vi "ParamScanSubVI.vi"(7 "Variable Cluster":T1={"Values"=[105.34210526315789, 210.5842105263158, 315.8263157894737, 421.0684210526316, 26.410526315789475, 131.65263157894736, 236.89473684210526, 342.1368421052632, 447.3789473684211, 52.72105263157895, 157.96315789473684, 263.20526315789476, 368.44736842105266, 473.68947368421055, 79.03157894736842, 184.2736842105263, 289.5157894736842, 394.7578947368421, 500.0], "Action"=20, "Inst."=0, "# Elements"=20, "Next Element"=6, "First Val"=0.1, "Final Val"=500.0, "Update Array"=FALSE, "Description"="relax", "Variable Type"=0, "Scan Now"=FALSE, "# Act/Inst."=11, "Electrodes_range"=[], "Parameter Name"="RW frequency (Hz)", "# Passes"=4} {"Variable Type" items=["Duration (s)", "Voltage (V)", "Parameter"]; "Final Val" format="%_6p"; "First Val" format="%_6p"; "Values" format="%_6p"}, 8 "Actions in":T4=[{"Toggle"=TRUE, "Open parameter editor"=FALSE, "Open MacroEditor"=FALSE, "Macro path"=path "", "Duration (s)"=2.0, "Parameters"=[{"Status"="Camera", "Name"="state (0,1)", "Value"=0.0, "Changed"=FALSE}, {"Status"="Slave", "Name"="state (0,1)", "Value"=0.0, "Changed"=FALSE}, {"Status"="Wait", "Name"="inbit (0...7)", "Value"=0.0, "Changed"=FALSE}, {"Status"="Coils", "Name"="buncher (A)", "Value"=10.0, "Changed"=TRUE}, {"Status"="Coils", "Name"="exit (A)", "Value"=25.0, "Changed"=TRUE}, {"Status"="Coils", "Name"="source (A)", "Value"=0.0, "Changed"=FALSE}, {"Status"="Coils", "Name"="stacker (A)", "Value"=0.0, "Changed"=FALSE}, {"Status"="Coils", "Name"="trans2 (A)", "Value"=0.0, "Changed"=FALSE}, {"Status"="Coils", "Name"="trans3 (A)", "Value"=0.0, "Changed"=FALSE}, {"Status"="Coils", "Name"="trans4 (A)", "Value"=0.0, "Changed"=FALSE}, {"Status"="RW", "Name"="mode (0-9)", "Value"=0.0, "Changed"=FALSE}, {"Status"="RW", "Name"="f_start (Hz)", "Value"=0.0, "Changed"=FALSE}, {"Status"="RW", "Name"="f_stop (Hz)", "Value"=0.0, "Changed"=FALSE}, {"Status"="RW", "Name"="amplitude (V)", "Value"=0.0, "Changed"=FALSE}, {"Status"="RW", "Name"="phase dif (deg)", "Value"=0.0, "Changed"=FALSE}, {"Status"="RW", "Name"="sweep time (s)", "Value"=0.0, "Changed"=FALSE}, {"Status"="HVpuls1", "Name"="enable (0,1)", "Value"=0.0, "Changed"=FALSE}, {"Status"="HVpuls1", "Name"="amplitude (V)", "Value"=0.0, "Changed"=FALSE}, {"Status"="HVpuls2", "Name"="enable (0,1)", "Value"=0.0, "Changed"=FALSE}, {"Status"="HVpuls2", "Name"="amplitude (V)", "Value"=0.0, "Changed"=FALSE}, {"Status"="HVpuls3", "Name"="enable (0,1)", "Value"=0.0, "Changed"=FALSE}, {"Status"="HVpuls3", "Name"="amplitude (V)", "Value"=0.0, "Changed"=FALSE}, {"Status"="MCP", "Name"="front bias (V)", "Value"=0.0, "Changed"=FALSE}, {"Status"="MCP", "Name"="back bias (V)", "Value"=0.0, "Changed"=FALSE}, {"Status"="MCP", "Name"="phos bias (V)", "Value"=0.0, "Changed"=FALSE}], "Comment"="buncher and exit on", "Reps"=1}, {"Toggle"=TRUE, "Open parameter editor"=FALSE, "Open MacroEditor"=FALSE, "Macro path"=path "", "Duration (s)"=0.1, "Parameters"=[{"Status"="Camera", "Name"="state (0,1)", "Value"=0.0, "Changed"=FALSE}, {"Status"="Slave", "Name"="state (0,1)", "Value"=0.0, "Changed"=FALSE}, {"Status"="Wait", "Name"="inbit (0...7)", "Value"=0.0, "Changed"=FALSE}, {"Status"="Coils", "Name"="buncher (A)", "Value"=0.0, "Changed"=TRUE}, {"Status"="Coils", "Name"="exit (A)", "Value"=0.0, "Changed"=TRUE}, {"Status"="Coils", "Name"="source (A)", "Value"=0.0, "Changed"=FALSE}, {"Status"="Coils", "Name"="stacker (A)", "Value"=0.0, "Changed"=FALSE}, {"Status"="Coils", "Name"="trans2 (A)", "Value"=0.0, "Changed"=FALSE}, {"Status"="Coils", "Name"="trans3 (A)", "Value"=0.0, "Changed"=FALSE}, {"Status"="Coils", "Name"="trans4 (A)", "Value"=0.0, "Changed"=FALSE}, {"Status"="RW", "Name"="mode (0-9)", "Value"=0.0, "Changed"=FALSE}, {"Status"="RW", "Name"="f_start (Hz)", "Value"=0.0, "Changed"=FALSE}, {"Status"="RW", "Name"="f_stop (Hz)", "Value"=0.0, "Changed"=FALSE}, {"Status"="RW", "Name"="amplitude (V)", "Value"=0.0, "Changed"=FALSE}, {"Status"="RW", "Name"="phase dif (deg)", "Value"=0.0, "Changed"=FALSE}, {"Status"="RW", "Name"="sweep time (s)", "Value"=0.0, "Changed"=FALSE}, {"Status"="HVpuls1", "Name"="enable (0,1)", "Value"=0.0, "Changed"=FALSE}, {"Status"="HVpuls1", "Name"="amplitude (V)", "Value"=0.0, "Changed"=FALSE}, {"Status"="HVpuls2", "Name"="enable (0,1)", "Value"=0.0, "Changed"=FALSE}, {"Status"="HVpuls2", "Name"="amplitude (V)", "Value"=0.0, "Changed"=FALSE}, {"Status"="HVpuls3", "Name"="enable (0,1)", "Value"=0.0, "Changed"=FALSE}, {"Status"="HVpuls3", "Name"="amplitude (V)", "Value"=0.0, "Changed"=FALSE}, {"Status"="MCP", "Name"="front bias (V)", "Value"=0.0, "Changed"=FALSE}, {"Status"="MCP", "Name"="back bias (V)", "Value"=0.0, "Changed"=FALSE}, {"Status"="MCP", "Name"="phos bias (V)", "Value"=0.0, "Changed"=FALSE}], "Comment"="off", "Reps"=1}] {"Reps" min=1 step=1; "Parameters"."Value" format="%_6p"; "Duration (s)" min=0.001 step=0.001 format="%_6p"}, 9 "Macro Info 2D in":T2(array[cluster])=[[{"Duration (s)"=2.0, "Instruction Description"="buncher and exit on", "Input Bits"=[], "Output Bits"=[FALSE, FALSE, FALSE, FALSE, FALSE, FALSE, FALSE, FALSE, FALSE, FALSE, FALSE, FALSE, FALSE, FALSE, FALSE, FALSE, FALSE, FALSE, FALSE, FALSE, FALSE, FALSE, FALSE, FALSE, FALSE, FALSE, FALSE, FALSE, FALSE, FALSE, FALSE, FALSE, FALSE, FALSE, FALSE, FALSE, FALSE, FALSE], "Excitations"=[0.0, 0.0, 0.0, 0.0, 0.0, 0.0, 0.0, 0.0, 0.0, 0.0, 0.0, 0.0, 0.0, 0.0, 0.0, 0.0, 0.0, 0.0, 0.0, 0.0, 0.0, 0.0, 0.0, 0.0], "Steps"=1, "Changes"=[TRUE, TRUE]}], [{"Duration (s)"=0.1, "Instruction Description"="off", "Input Bits"=[], "Output Bits"=[FALSE, FALSE, FALSE, FALSE, FALSE, FALSE, FALSE, FALSE, FALSE, FALSE, FALSE, FALSE, FALSE, FALSE, FALSE, FALSE, FALSE, FALSE, FALSE, FALSE, FALSE, FALSE, FALSE, FALSE, FALSE, FALSE, FALSE, FALSE, FALSE, FALSE, FALSE, FALSE, FALSE, FALSE, FALSE, FALSE, FALSE, FALSE], "Excitations"=[0.0, 0.0, 0.0, 0.0, 0.0, 0.0, 0.0, 0.0, 0.0, 0.0, 0.0, 0.0, 0.0, 0.0, 0.0, 0.0, 0.0, 0.0, 0.0, 0.0, 0.0, 0.0, 0.0, 0.0], "Steps"=1, "Changes"=[TRUE, TRUE]}]], 10 "# always zero":i32, 11 "Calibrations":T3=[{"Gain"=15.0098, "Offset (V)"=0.0035, "Name"="Vm"}, {"Gain"=14.9932, "Offset (V)"=0.0066, "Name"="in"}, {"Gain"=14.9651, "Offset (V)"=0.0072, "Name"="s1"}, {"Gain"=14.9843, "Offset (V)"=0.0049, "Name"="s2"}, {"Gain"=14.9433, "Offset (V)"=0.0056, "Name"="s3"}, {"Gain"=14.9395, "Offset (V)"=0.0041, "Name"="s4"}, {"Gain"=14.8775, "Offset (V)"=0.006, "Name"="g8"}, {"Gain"=14.9361, "Offset (V)"=0.0045, "Name"="--"}, {"Gain"=15.1086, "Offset (V)"=0.0054, "Name"="e1"}, {"Gain"=14.9264, "Offset (V)"=0.0039, "Name"="c1"}, {"Gain"=14.8685, "Offset (V)"=0.0066, "Name"="c2"}, {"Gain"=14.9386, "Offset (V)"=0.0045, "Name"="c3"}, {"Gain"=14.9438, "Offset (V)"=0.0032, "Name"="c4"}, {"Gain"=14.93, "Offset (V)"=0.0052, "Name"="c5"}, {"Gain"=14.9119, "Offset (V)"=0.0093, "Name"="c6"}, {"Gain"=14.9135, "Offset (V)"=0.0055, "Name"="c7"}, {"Gain"=14.9961, "Offset (V)"=0.0148, "Name"="c8"}, {"Gain"=14.9315, "Offset (V)"=0.0024, "Name"="c9"}, {"Gain"=14.9245, "Offset (V)"=0.006, "Name"="e2"}, {"Gain"=14.9016, "Offset (V)"=0.0037, "Name"="--"}, {"Gain"=14.9057, "Offset (V)"=0.0055, "Name"="--"}, {"Gain"=14.9213, "Offset (V)"=0.004, "Name"="--"}, {"Gain"=14.8995, "Offset (V)"=0.0013, "Name"="--"}, {"Gain"=14.9373, "Offset (V)"=0.004, "Name"="--"}] {"Offset (V)" format="%_6p"; "Gain" format="%_6p"}) -> (0 "Actions out":T4=[{"Toggle"=TRUE, "Open parameter editor"=FALSE, "Open MacroEditor"=FALSE, "Macro path"=path "", "Duration (s)"=2.0, "Parameters"=[{"Status"="Camera", "Name"="state (0,1)", "Value"=0.0, "Changed"=FALSE}, {"Status"="Slave", "Name"="state (0,1)", "Value"=0.0, "Changed"=FALSE}, {"Status"="Wait", "Name"="inbit (0...7)", "Value"=0.0, "Changed"=FALSE}, {"Status"="Coils", "Name"="buncher (A)", "Value"=10.0, "Changed"=TRUE}, {"Status"="Coils", "Name"="exit (A)", "Value"=30.0, "Changed"=TRUE}, {"Status"="Coils", "Name"="source (A)", "Value"=0.0, "Changed"=FALSE}, {"Status"="Coils", "Name"="stacker (A)", "Value"=0.0, "Changed"=FALSE}, {"Status"="Coils", "Name"="trans2 (A)", "Value"=0.0, "Changed"=FALSE}, {"Status"="Coils", "Name"="trans3 (A)", "Value"=0.0, "Changed"=FALSE}, {"Status"="Coils", "Name"="trans4 (A)", "Value"=0.0, "Changed"=FALSE}, {"Status"="RW", "Name"="mode (0-9)", "Value"=0.0, "Changed"=FALSE}, {"Status"="RW", "Name"="f_start (Hz)", "Value"=0.0, "Changed"=FALSE}, {"Status"="RW", "Name"="f_stop (Hz)", "Value"=0.0, "Changed"=FALSE}, {"Status"="RW", "Name"="amplitude (V)", "Value"=0.0, "Changed"=FALSE}, {"Status"="RW", "Name"="phase dif (deg)", "Value"=0.0, "Changed"=FALSE}, {"Status"="RW", "Name"="sweep time (s)", "Value"=0.0, "Changed"=FALSE}, {"Status"="HVpuls1", "Name"="enable (0,1)", "Value"=0.0, "Changed"=FALSE}, {"Status"="HVpuls1", "Name"="amplitude (V)", "Value"=0.0, "Changed"=FALSE}, {"Status"="HVpuls2", "Name"="enable (0,1)", "Value"=0.0, "Changed"=FALSE}, {"Status"="HVpuls2", "Name"="amplitude (V)", "Value"=0.0, "Changed"=FALSE}, {"Status"="HVpuls3", "Name"="enable (0,1)", "Value"=0.0, "Changed"=FALSE}, {"Status"="HVpuls3", "Name"="amplitude (V)", "Value"=0.0, "Changed"=FALSE}, {"Status"="MCP", "Name"="front bias (V)", "Value"=0.0, "Changed"=FALSE}, {"Status"="MCP", "Name"="back bias (V)", "Value"=0.0, "Changed"=FALSE}, {"Status"="MCP", "Name"="phos bias (V)", "Value"=0.0, "Changed"=FALSE}], "Comment"="buncher and exit on", "Reps"=1}, {"Toggle"=TRUE, "Open parameter editor"=FALSE, "Open MacroEditor"=FALSE, "Macro path"=path "", "Duration (s)"=0.1, "Parameters"=[{"Status"="Camera", "Name"="state (0,1)", "Value"=0.0, "Changed"=FALSE}, {"Status"="Slave", "Name"="state (0,1)", "Value"=0.0, "Changed"=FALSE}, {"Status"="Wait", "Name"="inbit (0...7)", "Value"=0.0, "Changed"=FALSE}, {"Status"="Coils", "Name"="buncher (A)", "Value"=0.0, "Changed"=TRUE}, {"Status"="Coils", "Name"="exit (A)", "Value"=0.0, "Changed"=TRUE}, {"Status"="Coils", "Name"="source (A)", "Value"=0.0, "Changed"=FALSE}, {"Status"="Coils", "Name"="stacker (A)", "Value"=0.0, "Changed"=FALSE}, {"Status"="Coils", "Name"="trans2 (A)", "Value"=0.0, "Changed"=FALSE}, {"Status"="Coils", "Name"="trans3 (A)", "Value"=0.0, "Changed"=FALSE}, {"Status"="Coils", "Name"="trans4 (A)", "Value"=0.0, "Changed"=FALSE}, {"Status"="RW", "Name"="mode (0-9)", "Value"=0.0, "Changed"=FALSE}, {"Status"="RW", "Name"="f_start (Hz)", "Value"=0.0, "Changed"=FALSE}, {"Status"="RW", "Name"="f_stop (Hz)", "Value"=0.0, "Changed"=FALSE}, {"Status"="RW", "Name"="amplitude (V)", "Value"=0.0, "Changed"=FALSE}, {"Status"="RW", "Name"="phase dif (deg)", "Value"=0.0, "Changed"=FALSE}, {"Status"="RW", "Name"="sweep time (s)", "Value"=0.0, "Changed"=FALSE}, {"Status"="HVpuls1", "Name"="enable (0,1)", "Value"=0.0, "Changed"=FALSE}, {"Status"="HVpuls1", "Name"="amplitude (V)", "Value"=0.0, "Changed"=FALSE}, {"Status"="HVpuls2", "Name"="enable (0,1)", "Value"=0.0, "Changed"=FALSE}, {"Status"="HVpuls2", "Name"="amplitude (V)", "Value"=0.0, "Changed"=FALSE}, {"Status"="HVpuls3", "Name"="enable (0,1)", "Value"=0.0, "Changed"=FALSE}, {"Status"="HVpuls3", "Name"="amplitude (V)", "Value"=0.0, "Changed"=FALSE}, {"Status"="MCP", "Name"="front bias (V)", "Value"=0.0, "Changed"=FALSE}, {"Status"="MCP", "Name"="back bias (V)", "Value"=0.0, "Changed"=FALSE}, {"Status"="MCP", "Name"="phos bias (V)", "Value"=0.0, "Changed"=FALSE}], "Comment"="off", "Reps"=1}] {"Reps" min=1 step=1; "Parameters"."Value" format="%_6p"; "Duration (s)" min=0.001 step=0.001 format="%_6p"}, 1 "Macro Info 2D out":T2(array[cluster])=[[{"Duration (s)"=2.0, "Instruction Description"="buncher and exit on", "Input Bits"=[], "Output Bits"=[FALSE, FALSE, FALSE, FALSE, FALSE, FALSE, FALSE, FALSE, FALSE, FALSE, FALSE, FALSE, FALSE, FALSE, FALSE, FALSE, FALSE, FALSE, FALSE, FALSE, FALSE, FALSE, FALSE, FALSE, FALSE, FALSE, FALSE, FALSE, FALSE, FALSE, FALSE, FALSE, FALSE, FALSE, FALSE, FALSE, FALSE, FALSE], "Excitations"=[0.0, 0.0, 0.0, 0.0, 0.0, 0.0, 0.0, 0.0, 0.0, 0.0, 0.0, 0.0, 0.0, 0.0, 0.0, 0.0, 0.0, 0.0, 0.0, 0.0, 0.0, 0.0, 0.0, 0.0], "Steps"=1, "Changes"=[TRUE, TRUE]}], [{"Duration (s)"=0.1, "Instruction Description"="off", "Input Bits"=[], "Output Bits"=[FALSE, FALSE, FALSE, FALSE, FALSE, FALSE, FALSE, FALSE, FALSE, FALSE, FALSE, FALSE, FALSE, FALSE, FALSE, FALSE, FALSE, FALSE, FALSE, FALSE, FALSE, FALSE, FALSE, FALSE, FALSE, FALSE, FALSE, FALSE, FALSE, FALSE, FALSE, FALSE, FALSE, FALSE, FALSE, FALSE, FALSE, FALSE], "Excitations"=[0.0, 0.0, 0.0, 0.0, 0.0, 0.0, 0.0, 0.0, 0.0, 0.0, 0.0, 0.0, 0.0, 0.0, 0.0, 0.0, 0.0, 0.0, 0.0, 0.0, 0.0, 0.0, 0.0, 0.0], "Steps"=1, "Changes"=[TRUE, TRUE]}]])   [LabVIEW 2018]
uses:
  QBuilder Files/Actions_arr.ctl
  QBuilder Files/Action.ctl
  QBuilder Files/Parameters.ctl
  Calibrations.ctl
  VariableScan_Cluster.ctl
panel:
  # "browse"
  # "browse"
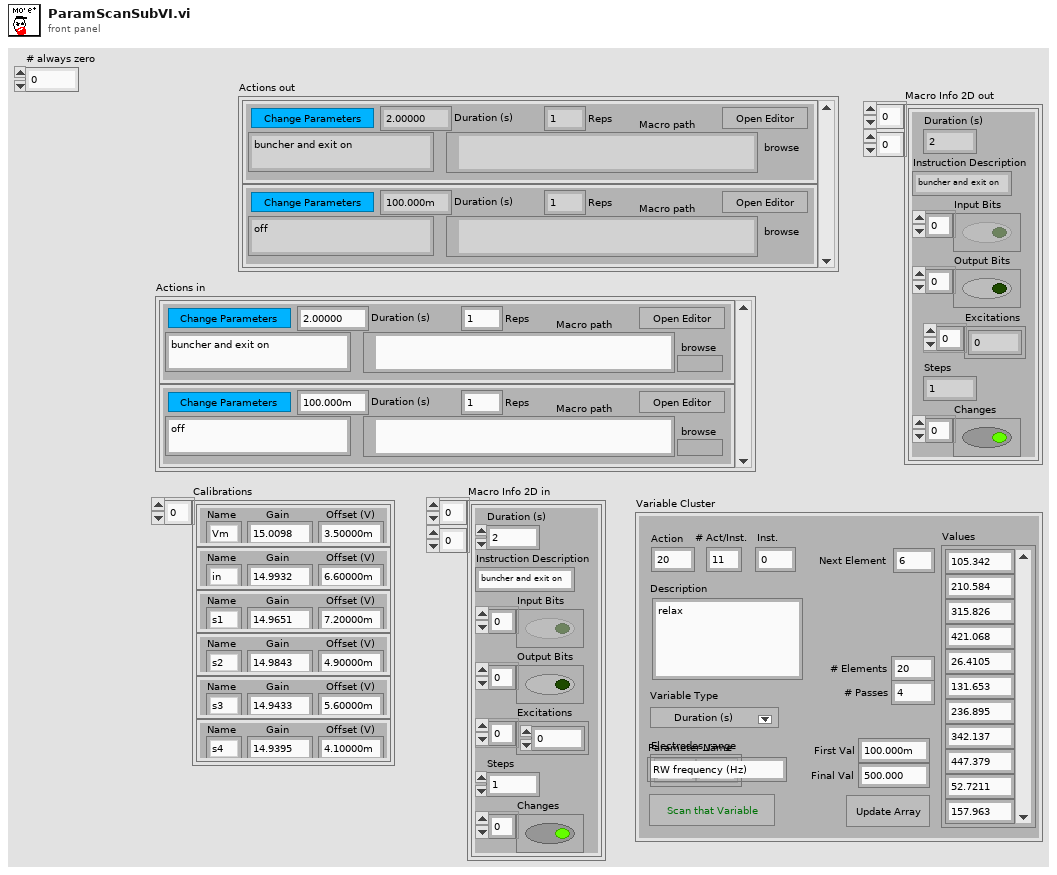
[diagram p1: front panel]
types:
  T1 = typedef "VariableScan_Cluster.ctl" = cluster{"Values":dbl[], "Action":i32, "Inst.":i32, "# Elements":i32, "Next Element":i32, "First Val":dbl, "Final Val":dbl, "Update Array":bool, "Description":string, "Variable Type":u16, "Scan Now":bool, "# Act/Inst.":i32, "Electrodes_range":i32[], "Parameter Name":string, "# Passes":i32}
  T2 = cluster{"Duration (s)":dbl, "Instruction Description":string, "Input Bits":bool[], "Output Bits":bool[], "Excitations":dbl[], "Steps":i32, "Changes":bool[]}[][]
  T3 = typedef "Calibrations.ctl" = cluster{"Gain":dbl, "Offset (V)":dbl, "Name":string}[]
  T4 = typedef "Actions_arr.ctl" = T5[]
  T5 = typedef "Action.ctl" = cluster{"Toggle":bool, "Open parameter editor":bool, "Open MacroEditor":bool, "Macro path":path, "Duration (s)":dbl, "Parameters":T6, "Comment":string, "Reps":i32}
  T6 = typedef "Parameters.ctl" = cluster{"Status":string, "Name":string, "Value":dbl, "Changed":bool}[]
  T7 = cluster{"Duration (s)":dbl, "Instruction Description":string, "Input Bits":bool[], "Output Bits":bool[], "Excitations":dbl[], "Steps":i32, "Changes":bool[]}
  T8 = cluster{"Status":string, "Name":string, "Value":dbl, "Changed":bool}
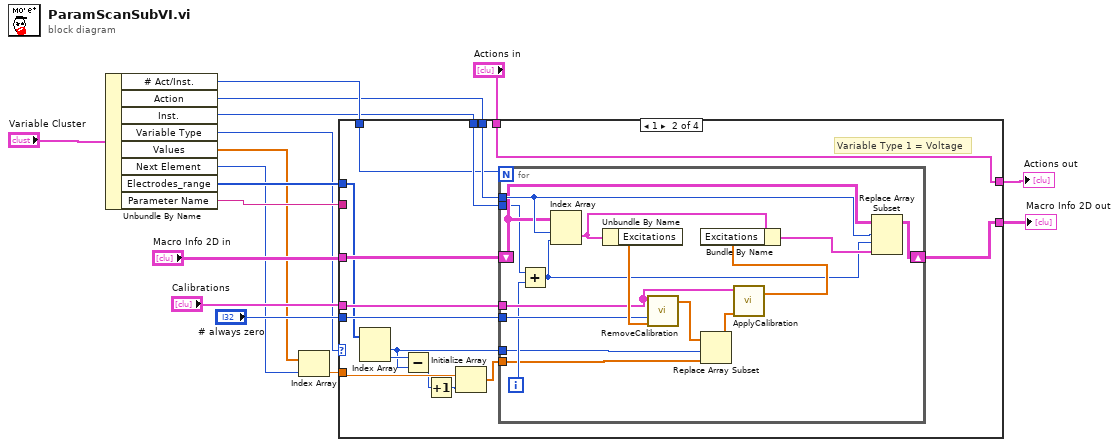
[diagram p0: block diagram]
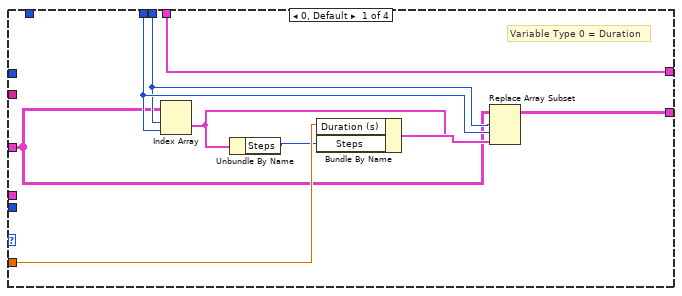
[diagram p2: hidden frame]
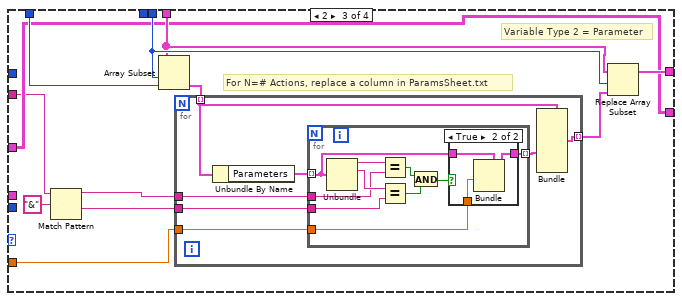
[diagram p3: hidden frame]
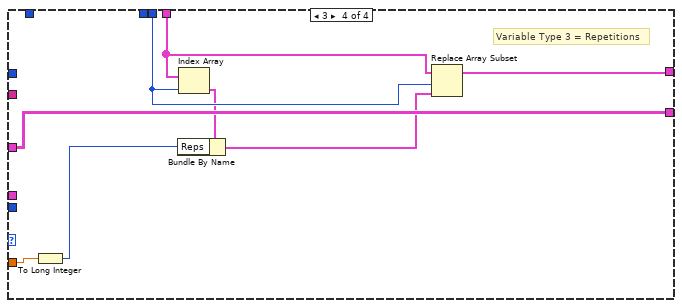
[diagram p5: hidden frame]
diagram:
  n1 = Unbundle By Name("Variable Cluster") -> ("# Act/Inst."=w8:i32, "Action"=w3:i32, "Inst."=w4:i32, "Variable Type"=w6:u16, "Values"=w7:dbl[], "Next Element"=w1:i32, "Electrodes_range"=w10:i32[], "Parameter Name"=w9:string)
  n2 = Index Array(array=w7, index=w1) -> (element=w5:dbl)
  n3 = case shown="1" w6 {
    tunnel: w3 -> [w22 w40 w68 w94]
    tunnel: w4 -> [w25 w39 _ _]
    tunnel: w5 -> [w21 w32 w57 w97]
    tunnel: w8 -> [_ w33 w65 _]
    tunnel: w9 -> [_ _ w60 _]
    tunnel: w10 -> [_ w30 _ _]
    tunnel: "Macro Info 2D in" -> [w19 w37 w62 w96]
    tunnel: [w18 w38 w62 w96] -> w12
    tunnel: "Calibrations" -> [_ w36 _ _]
    tunnel: "# always zero" -> [_ w35 _ _]
    tunnel: "Actions in" -> [w17 w34 w64 w95]
    tunnel: [w17 w34 w63 w90] -> w16
    frame 0, Default {
      # "Variable Type 0 = Duration"
      n4 = Index Array(array=w19, index (row)=w22, index (col)=w25) -> (element=w23:T7)
      n5 = Unbundle By Name(w23) -> ("Steps"=w20:i32)
      n6 = Bundle By Name(cluster=w23, "Duration (s)"=w21, "Steps"=w20) -> (w24:T7)
      n7 = Replace Array Subset(array=w19, new element=w24, index (row)=w22, index (col)=w25) -> (w18:T2)
    }
    frame 1 {
      # "Variable Type 1 = Voltage"
      n8 = Index Array(array=w30) -> (element #1=w28:i32, element #2=w29:i32)  [unwired: 2 in]
      n9 = Subtract(x=w29, y=w28) -> (x-y=w27:i32)
      n10 = Increment(x=w27) -> (x+1=w26:i32)
      n11 = Initialize Array(w32, w26) -> (w31:dbl[])
      n12 = for {
        N: w33 -> [_]
        tunnel: w40 -> [w55]
        tunnel: w39 -> [w45]
        tunnel: w36 -> [w47]
        tunnel: w35 -> [w46]
        shift-right: [w49] -> w38
        shift-left: w37 -> [w48]
        tunnel: w31 -> [w42]
        tunnel: w28 -> [w41]
        i -> [w44]
        n13 = Add(x=w45, y=w44) -> (x+y=w43:i32)
        n14 = Index Array(array=w48, index (row)=w55, index (col)=w43) -> (element=w56:T7)
        n15 = Unbundle By Name(w56) -> ("Excitations"=w53:dbl[])
        n16 = call "RemoveCalibration.vi"("Excitations"=w53, "# always zero"=w46, "Calibrations"=w47) -> ("Potentials"=w52:dbl[])  [unwired: 2 in]
        n17 = Replace Array Subset(array=w52, new element=w42, index=w41) -> (w51:dbl[])
        n18 = call "ApplyCalibration.vi"("Potentials"=w51, "Calibrations"=w47) -> ("Excitations"=w50:dbl[])  [unwired: 2 in, 1 out]
        n19 = Bundle By Name(cluster=w56, "Excitations"=w50) -> (w54:T7)
        n20 = Replace Array Subset(array=w48, new element=w54, index (row)=w55, index (col)=w43) -> (w49:T2)
      }
    }
    frame 2 {
      # "For N=# Actions, replace a column in ParamsSheet.txt"
      # "Variable Type 2 = Parameter"
      n21 = Match Pattern(string=w60, regular expression="&") -> (before substring=w59:string, after substring=w58:string)  [unwired: 1 in, 2 out]
      n22 = Array Subset(array=w64, index=w68, length=w65) -> (w67:T4)
      n23 = for {
        tunnel: w57 -> [w75]
        tunnel: w67 -> [w72] mode=indexing
        tunnel: [w71] -> w66 mode=indexing
        tunnel: w59 -> [w70]
        tunnel: w58 -> [w69]
        n24 = Unbundle By Name(w72) -> ("Parameters"=w73:T6)
        n25 = for {
          tunnel: w73 -> [w85] mode=indexing
          tunnel: [w84] -> w74 mode=indexing
          tunnel: w75 -> [w83]
          tunnel: w70 -> [w77]
          tunnel: w69 -> [w76]
          n26 = Unbundle(w85) -> ("Status"=w82:string, "Name"=w81:string)  [unwired: 2 out]
          n27 = Equal?(x=w82, y=w77) -> (x = y?=w79:bool)
          n28 = Equal?(x=w81, y=w76) -> (x = y?=w78:bool)
          n29 = And(x=w79, y=w78) -> (x .and. y?=w80:bool)
          n30 = case shown="True" w80 {
            tunnel: w85 -> [w86 w89]
            tunnel: [w86 w88] -> w84
            tunnel: w83 -> [_ w87]
            frame False {
            }
            frame True {
              n31 = Bundle(cluster=w89, "Value"=w87) -> (w88:T8)  [unwired: 3 in]
            }
          }
        }
        n32 = Bundle(cluster=w72, "Parameters"=w74) -> (w71:T5)  [unwired: 7 in]
      }
      n33 = Replace Array Subset(array=w64, new element=w66, index=w68) -> (w63:T4)
    }
    frame 3 {
      # "Variable Type 3 = Repetitions"
      n34 = To Long Integer(number=w97) -> (32bit integer=w92:i32)
      n35 = Index Array(array=w95, index=w94) -> (element=w93:T5)
      n36 = Bundle By Name(cluster=w93, "Reps"=w92) -> (w91:T5)
      n37 = Replace Array Subset(array=w95, new element=w91, index=w94) -> (w90:T4)
    }
  }
  "Actions out" <- w16
  "Macro Info 2D out" <- w12
